vi "Read_Temperatures.vi"(8 "error in (no error)":errorcluster, 11 "USB-87Pn_Data In":T1) -> (0 "error out":errorcluster, 2 "Temperature Data":sgl[][](array[numeric]), 3 "USB-87Pn_Data Out":T1)   [LabVIEW 2019, in "USB-87P8_Manager.lvlib"]
uses:
  Module/USB-87P8_Manager.lvlib
  USB-87Pn_Data.ctl
  USB-87Pn.lvclass
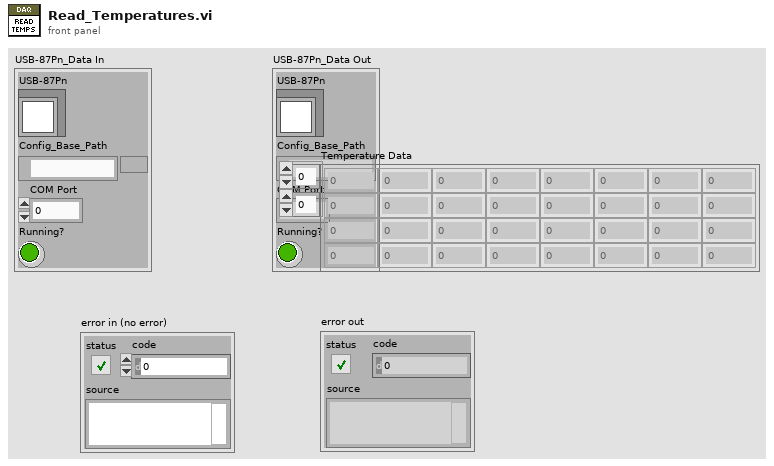
[diagram p1: front panel]
types:
  T1 = typedef "USB-87P8_Manager.lvlib/USB-87Pn_Data.ctl" = cluster{"USB-87Pn":refnum<class "USB-87Pn.lvclass">, "Config_Base_Path":path, "COM Port":i32, "Running?":bool}
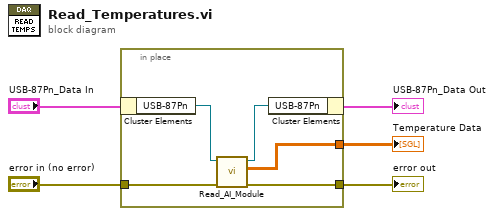
[diagram p0: block diagram]
diagram:
  n1 = in-place {
    in-place-border: "error in (no error)" -> [w10]
    in-place-border: [w9] -> w4
    in-place-border: [w6] -> w1
    n2 = in-place-cluster #1("USB-87Pn_Data In") -> ("USB-87Pn"=w8:refnum<class "USB-87Pn.lvclass">)
    n3 = call "Read_AI_Module.vi"("error in (no error)"=w10, "USB-87Pn in"=w8) -> ("error out"=w9:errorcluster, "AI float"=w6:sgl[][], "USB-87Pn out"=w7:refnum<class "USB-87Pn.lvclass">)  [unwired: 7 in]
    n4 = in-place-cluster #1("USB-87Pn"=w7) -> (→"USB-87Pn_Data Out":T1)
  }
  "error out" <- w4
  "Temperature Data" <- w1
